vi "Digital Pattern Sim Test.vi"() -> ()   [LabVIEW 2015]
uses:
  IP Source/Digital Pattern Generation/Settings.ctl
  IP Source/Digital Pattern Generation/Load Input.ctl
  <vilib>/rvi/interface/RandomDataEmulation/nirviRandomDataOpen.vi
  <vilib>/rvi/interface/common/niFpgaCacheSessionInfoDynamic.vi
  <vilib>/Utility/error.llb/Error Cluster From Error Code.vi
  <vilib>/rvi/errors/niLvFpgaAdjustHostInterfaceError.vi
  <vilib>/FPGAPlugInAG/Dynamic/niLvFpga_Run_Dynamic.vi
  <vilib>/FPGAPlugInAG/Dynamic/niLvFpga_Close_Dynamic.vi
  <vilib>/rvi/interface/nirviOpenFPGA/nirviOpenFPGA.xnode
  Simulation FPGA/APU + Digital Pattern Sim.vi
  <vilib>/rvi/interface/nirviReadWriteControl/nirviReadWriteControl.xnode
  <vilib>/rvi/interface/nirviMethod/nirviMethod.xnode
  <vilib>/rvi/interface/nirviCloseFPGA/nirviCloseFPGA.xnode
  <vilib>/rvi/interface/Simulation/niFpgaSimulationCallBeginRW.vi
  IP Source/Digital Pattern Generation/Digital Pattern Generation.lvlib
  NiFpgaLv.dll
panel:
  in  "cycle angle":bool=TRUE
  in  "Tooth Angles":cluster{"Rising Edge":dbl, "Falling Edge":dbl}[](array[cluster])=[{"Rising Edge"=100.0, "Falling Edge"=200.0}, {"Rising Edge"=300.0, "Falling Edge"=400.0}]
  out "Load done":bool
  out "Load time (s)":dbl=2.001387469202996
  in  "Angle":dbl format="%#_15g"
  in  "stop":bool
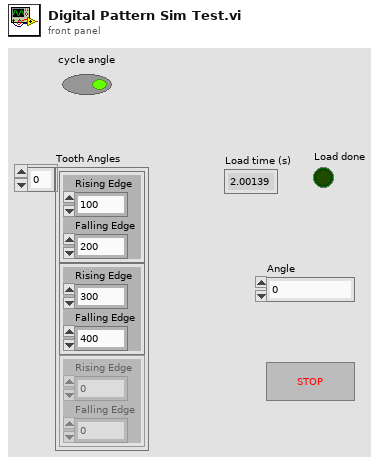
[diagram p1: front panel]
types:
  T1 = typedef "Engine Simulation Toolkit.lvlib/Digital Pattern Generation.lvlib/Settings.ctl" = cluster{"edge 1":u16, "edge 2":u16, "cycle angle":bool, "enabled":bool, "first falling":bool, "fault":bool, "fault wrap":bool, "fault value":bool, "fault count":fxp<+,4,4>, "use fault count":bool}
  T2 = typedef "Engine Simulation Toolkit.lvlib/Digital Pattern Generation.lvlib/Load Input.ctl" = cluster{"address":fxp<+,11,11>, "done":bool, "angle":u16}
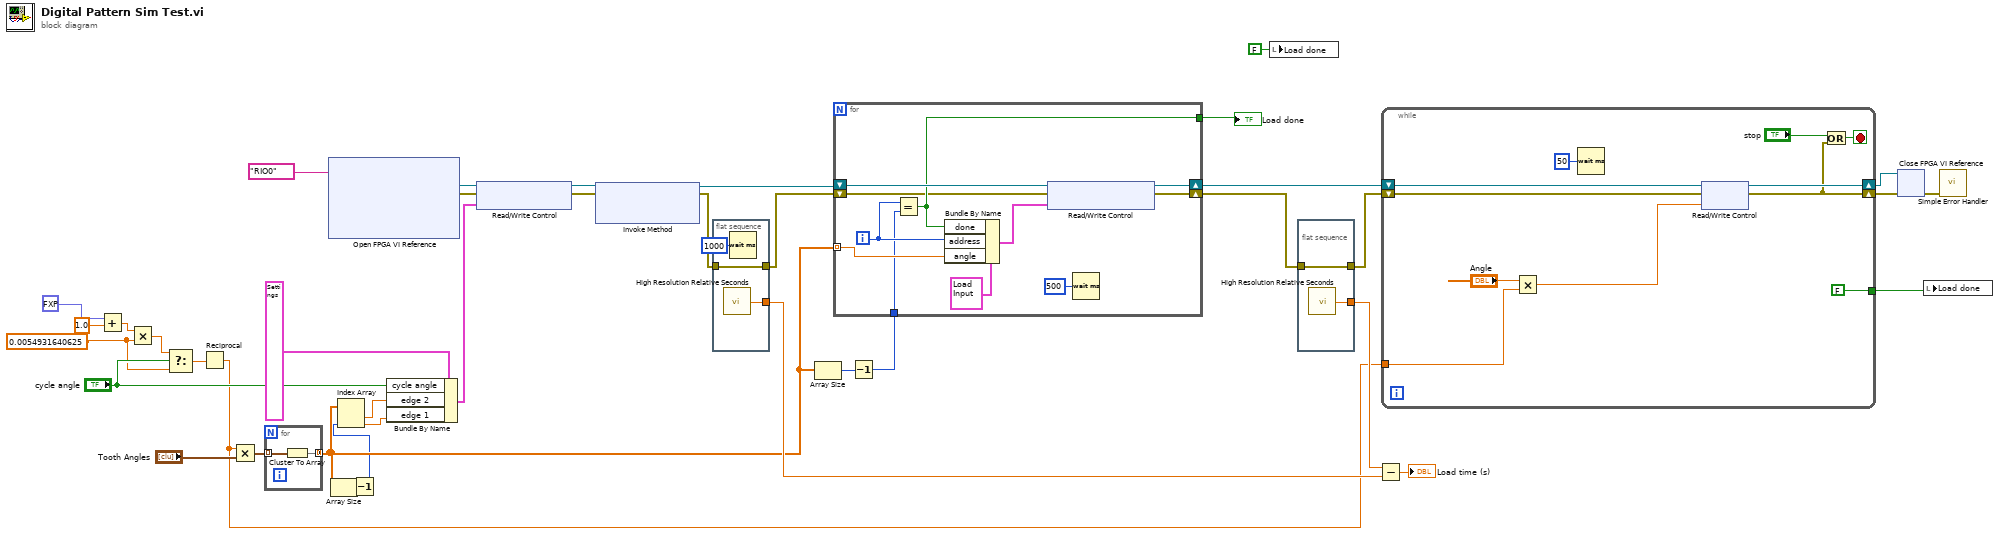
[diagram p0: block diagram]
diagram:
  w12 = 0.0054931640625 ("x")
  n1 = Add(x=fxp<+,2,2> 1.0 ("extra cranks for a cycle"), y=1.0) -> (x+y=w22:dbl)
  n2 = Multiply(x=w22, y=w12) -> (x*y=w14:dbl)
  n3 = Select(t=w14, s="cycle angle", f=w12) -> (s? t:f=w13:dbl)
  n4 = Reciprocal(x=w13) -> (1/x=w1:dbl)
  n5 = Multiply(x=w1, y="Tooth Angles") -> (x*y=w11:cluster{"Rising Edge":dbl, "Falling Edge":dbl}[])
  n6 = for {
    tunnel: w11 -> [w41] mode=indexing
    tunnel: [w40] -> w5 mode=concatenating
    n7 = Cluster To Array(cluster=w41) -> (array=w40:dbl[])
  }
  n8 = xnode "Open FPGA VI Reference"("resource name"=tag "RIO0") -> ("FPGA VI Reference Out"=w6:refnum<k20>, "error out"=w36:errorcluster)  [unwired: 1 in]
  n9 = Array Size(array=w5) -> (size(s)=w4:i32)
  n10 = Decrement(x=w4) -> (x-1=w2:i32)
  n11 = Index Array(array=w5, index #2=w2) -> (element #1=w7:dbl, element #2=w3:dbl)  [unwired: 1 in]
  n12 = Bundle By Name(cluster=T1 {"edge 1"=0, "edge 2"=0, "cycle angle"=TRUE, "enabled"=TRUE, "first falling"=FALSE, "fault"=FALSE, "fault wrap"=FALSE, "fault value"=FALSE, "fault count"=0.0, "use fault count"=FALSE} ("settings.<user name>"), "cycle angle"="cycle angle", "edge 2"=w7, "edge 1"=w3) -> (w16:T1)
  n13 = xnode "Read/Write Control"("FPGA VI Reference In"=w6, "error in"=w36, "settings.Pattern 1"=w16) -> ("FPGA VI Reference Out"=w20:refnum<k20>, "error out"=w21:errorcluster)
  n14 = xnode "Invoke Method"("FPGA VI Reference In"=w20, "error in"=w21) -> ("FPGA VI Reference Out"=w32:refnum<k20>, "error out"=w30:errorcluster)  [unwired: 1 in]
  n15 = flat-sequence {
    tunnel: [w44] -> w31
    tunnel: w30 -> [w44]
    tunnel: [w43] -> w28
    frame #0 {
      n16 = call <vilib>:"High Resolution Relative Seconds.vi"() -> ("relative seconds"=w43:dbl)
      n17 = Wait (ms)(milliseconds to wait=u32 1000) -> ()  [unwired: 1 out]
    }
  }
  n18 = Array Size(array=w5) -> (size(s)=w10:i32)
  n19 = Decrement(x=w10) -> (x-1=w9:i32)
  n20 = for {
    shift-right: [w52] -> w25
    shift-left: w31 -> [w45]
    shift-right: [w54] -> w26
    shift-left: w32 -> [w55]
    tunnel: w5 -> [w50] mode=indexing
    tunnel: w9 -> [w48]
    tunnel: [w46] -> w8
    i -> [w49]
    n21 = Equal?(x=w49, y=w48) -> (x = y?=w46:bool)
    n22 = Bundle By Name(cluster=T2 {"address"=0.0, "done"=FALSE, "angle"=0} ("load input.<user name>"), "done"=w46, "address"=w49, "angle"=w50) -> (w47:T2)
    n23 = xnode "Read/Write Control"("FPGA VI Reference In"=w55, "error in"=w45, "LoadInput.Pattern 1"=w47) -> ("FPGA VI Reference Out"=w54:refnum<k20>, "error out"=w52:errorcluster)
    n24 = Wait (ms)(milliseconds to wait=u32 500) -> ()  [unwired: 1 out]
  }
  "Load done" <- w8
  n25 = local write "Load done"(FALSE ("Load done")) -> ()
  n26 = flat-sequence {
    tunnel: [w57] -> w24
    tunnel: w25 -> [w57]
    tunnel: [w56] -> w29
    frame #0 {
      n27 = call <vilib>:"High Resolution Relative Seconds.vi"() -> ("relative seconds"=w56:dbl)
    }
  }
  n28 = Subtract(x=w29, y=w28) -> (x-y=→"Load time (s)":dbl)
  n29 = while {
    shift-right: [w63] -> w39
    shift-left: w24 -> [w68]
    shift-right: [w66] -> w38
    shift-left: w26 -> [w67]
    tunnel: [FALSE ("Load")] -> w34
    tunnel: w1 -> [w59]
    stop <- w64 stop-if-true
    n30 = Multiply(x="Angle", y=w59) -> (x*y=w58:dbl)
    n31 = Wait (ms)(milliseconds to wait=u32 50) -> ()  [unwired: 1 out]
    n32 = xnode "Read/Write Control"("FPGA VI Reference In"=w67, "error in"=w68, "Data"=w58) -> ("FPGA VI Reference Out"=w66:refnum<k20>, "error out"=w63:errorcluster)
    n33 = Or(x="stop", y=w63) -> (x .or. y?=w64:bool)
  }
  n34 = xnode "Close FPGA VI Reference"("FPGA VI Reference In"=w38, "error in"=w39) -> ("error out"=w37:errorcluster)
  n35 = local write "Load done"(w34) -> ()
  n36 = call <vilib>:"Simple Error Handler.vi"("error in (no error)"=w37) -> ()  [unwired: 4 in, 5 out]
